vi "serial del.vi"() -> ()   [LabVIEW 2014]
uses:
  <vilib>/Utility/sysdir.llb/System Directory Type.ctl
panel:
  in  "?":bool
  out "?":string
  in  "정규식":string
  in  "정규식 2":string
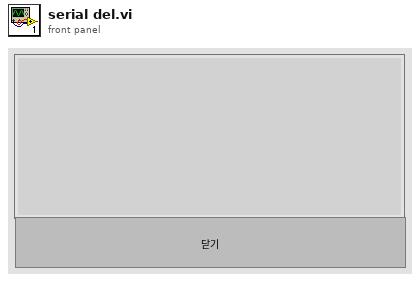
[diagram p1: front panel]
types:
  T1 = enum16{"open", "replace", "create", "open or create", "replace or create", "replace or create with confirmation"}
  T2 = typedef "System Directory Type.ctl" = i32
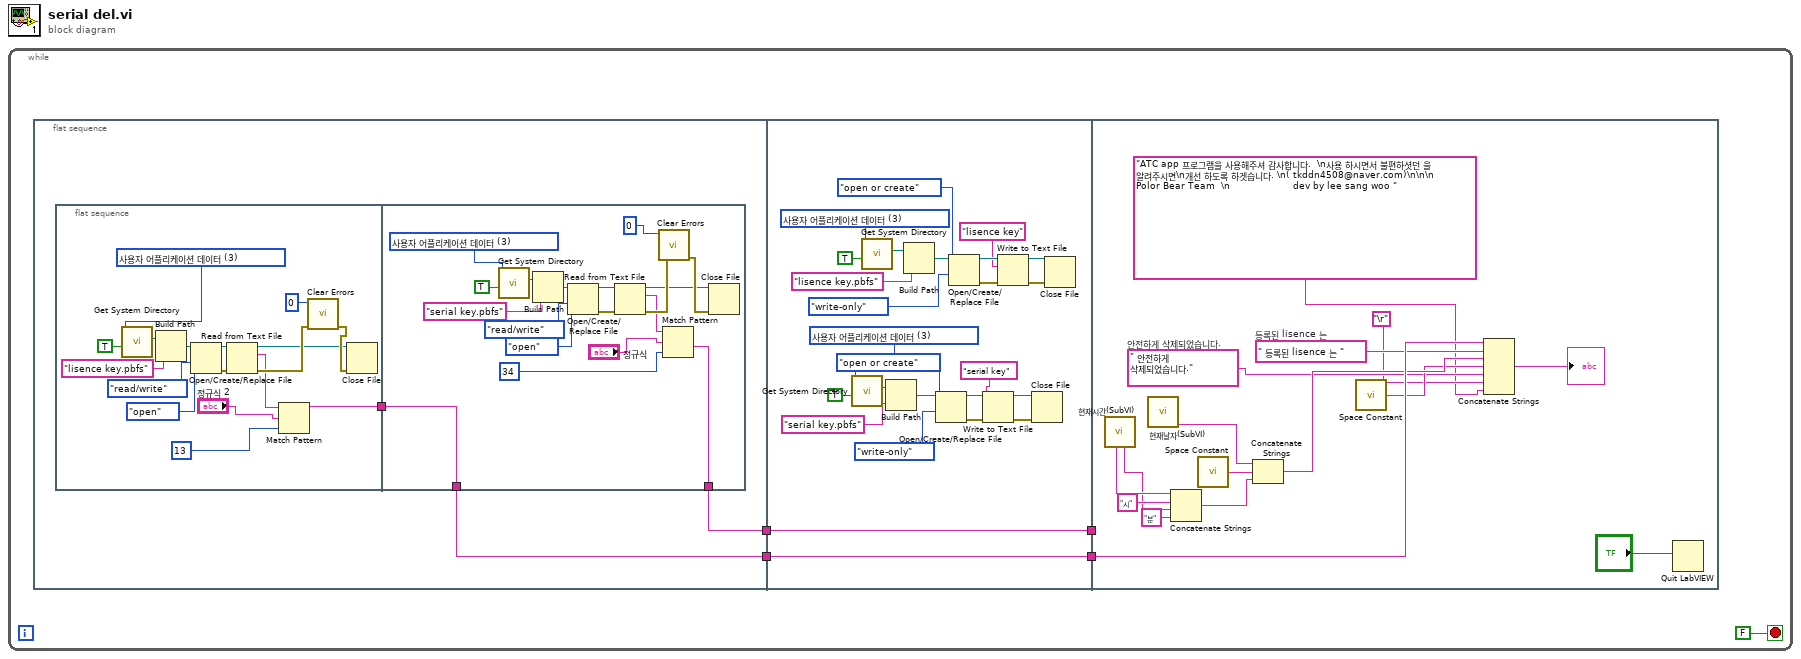
[diagram p0: block diagram]
diagram:
  n1 = while {
    stop <- FALSE stop-if-true
    n2 = flat-sequence {
      tunnel: [w7] -> w5
      tunnel: [w6] -> w4
      tunnel: w5 -> [w44]
      tunnel: [w45] -> w3
      tunnel: w4 -> [w45]
      tunnel: [w44] -> w2
      tunnel: w3 -> [w85]
      tunnel: w2 -> [_]
      frame #0 {
        n3 = flat-sequence {
          tunnel: [w10] -> w8
          tunnel: w8 -> [w27]
          tunnel: [w28] -> w7
          tunnel: [w27] -> w6
          frame #0 {
            w15 = T2 3 items=["사용자 홈"=0, "사용자 데스크탑"=1, "사용자 문서"=2, "사용자 어플리케이션 데이터"=3, "사용자 환경"=4, "사용자 임시"=5, "퍼블릭 문서"=6, "퍼블릭 어플리케이션 데이터"=7, "퍼블릭 환경"=8, "퍼블릭 캐시"=13, "시스템 코어 라이브러리"=9, "시스템 설치된 라이브러리"=10, "어플리케이션 파일"=11, "부팅 볼륨 루트"=12] ("system directory type")
            n4 = call <vilib>:"Get System Directory.vi"("create directory if not found? (F)"=TRUE, "system directory type"=w15) -> ("system directory"=w14:path)  [unwired: 9 in]
            n5 = Build Path(base path=w14, name or relative path="lisence key.pbfs" ("이름 또는 상대 경로")) -> (appended path=w13:path)
            n6 = Open/Create/Replace File(file path (use dialog)=w13, operation (0:open)=T1."open" ("동작(0:open)"), access (0:read/write)=enum16{"read/write", "read-only", "write-only"}."read/write" ("접근(0:읽기/쓰기)")) -> (refnum out=w19:refnum<file>, error out=w18:errorcluster)  [unwired: 3 in, 1 out]
            n7 = Read from Text File(file (use dialog)=w19, error in=w18) -> (refnum out=w20:refnum<file>, text=w21:string, error out=w23:errorcluster)  [unwired: 2 in, 1 out]
            n8 = Match Pattern(string=w21, regular expression="정규식 2", offset (0)=13 ("오프셋(0) 2")) -> (before substring=w10:string)  [unwired: 3 out]
            n9 = call <vilib>:"Clear Errors.vi"("error in (no error)"=w23, "specific error code to clear (0: all)"=0) -> ("error out"=w24:errorcluster)  [unwired: 4 in, 1 out]
            n10 = Close File(refnum=w20, error in=w24) -> ()  [unwired: 2 out]
          }
          frame #1 {
            w36 = T2 3 items=["사용자 홈"=0, "사용자 데스크탑"=1, "사용자 문서"=2, "사용자 어플리케이션 데이터"=3, "사용자 환경"=4, "사용자 임시"=5, "퍼블릭 문서"=6, "퍼블릭 어플리케이션 데이터"=7, "퍼블릭 환경"=8, "퍼블릭 캐시"=13, "시스템 코어 라이브러리"=9, "시스템 설치된 라이브러리"=10, "어플리케이션 파일"=11, "부팅 볼륨 루트"=12] ("system directory type")
            n11 = call <vilib>:"Get System Directory.vi"("create directory if not found? (F)"=TRUE, "system directory type"=w36) -> ("system directory"=w37:path)  [unwired: 9 in]
            n12 = Build Path(base path=w37, name or relative path="serial key.pbfs" ("이름 또는 상대 경로")) -> (appended path=w38:path)
            n13 = Open/Create/Replace File(file path (use dialog)=w38, operation (0:open)=T1."open" ("동작(0:open)"), access (0:read/write)=enum16{"read/write", "read-only", "write-only"}."read/write" ("접근(0:읽기/쓰기)")) -> (refnum out=w32:refnum<file>, error out=w33:errorcluster)  [unwired: 3 in, 1 out]
            n14 = Read from Text File(file (use dialog)=w32, error in=w33) -> (refnum out=w31:refnum<file>, text=w39:string, error out=w41:errorcluster)  [unwired: 2 in, 1 out]
            n15 = call <vilib>:"Clear Errors.vi"("error in (no error)"=w41, "specific error code to clear (0: all)"=0) -> ("error out"=w42:errorcluster)  [unwired: 4 in, 1 out]
            n16 = Match Pattern(string=w39, regular expression="정규식", offset (0)=34 ("오프셋(0)")) -> (after substring=w28:string)  [unwired: 3 out]
            n17 = Close File(refnum=w31, error in=w42) -> ()  [unwired: 2 out]
          }
        }
      }
      frame #1 {
        w53 = T2 3 items=["사용자 홈"=0, "사용자 데스크탑"=1, "사용자 문서"=2, "사용자 어플리케이션 데이터"=3, "사용자 환경"=4, "사용자 임시"=5, "퍼블릭 문서"=6, "퍼블릭 어플리케이션 데이터"=7, "퍼블릭 환경"=8, "퍼블릭 캐시"=13, "시스템 코어 라이브러리"=9, "시스템 설치된 라이브러리"=10, "어플리케이션 파일"=11, "부팅 볼륨 루트"=12] ("system directory type")
        w65 = T2 3 items=["사용자 홈"=0, "사용자 데스크탑"=1, "사용자 문서"=2, "사용자 어플리케이션 데이터"=3, "사용자 환경"=4, "사용자 임시"=5, "퍼블릭 문서"=6, "퍼블릭 어플리케이션 데이터"=7, "퍼블릭 환경"=8, "퍼블릭 캐시"=13, "시스템 코어 라이브러리"=9, "시스템 설치된 라이브러리"=10, "어플리케이션 파일"=11, "부팅 볼륨 루트"=12] ("system directory type")
        n18 = call <vilib>:"Get System Directory.vi"("create directory if not found? (F)"=TRUE, "system directory type"=w65) -> ("system directory"=w66:path)  [unwired: 9 in]
        n19 = call <vilib>:"Get System Directory.vi"("create directory if not found? (F)"=TRUE, "system directory type"=w53) -> ("system directory"=w52:path)  [unwired: 9 in]
        n20 = Build Path(base path=w66, name or relative path="serial key.pbfs" ("이름 또는 상대 경로")) -> (appended path=w67:path)
        n21 = Build Path(base path=w52, name or relative path="lisence key.pbfs" ("이름 또는 상대 경로")) -> (appended path=w51:path)
        n22 = Open/Create/Replace File(file path (use dialog)=w67, operation (0:open)=T1."open or create" ("동작(0:open)"), access (0:read/write)=enum16{"read/write", "read-only", "write-only"}."write-only" ("접근(0:읽기/쓰기)")) -> (refnum out=w60:refnum<file>, error out=w61:errorcluster)  [unwired: 3 in, 1 out]
        n23 = Open/Create/Replace File(file path (use dialog)=w51, operation (0:open)=T1."open or create" ("동작(0:open)"), access (0:read/write)=enum16{"read/write", "read-only", "write-only"}."write-only" ("접근(0:읽기/쓰기)")) -> (refnum out=w55:refnum<file>, error out=w56:errorcluster)  [unwired: 3 in, 1 out]
        n24 = Write to Text File(file (use dialog)=w60, text="serial key" ("이름 또는 상대 경로"), error in=w61) -> (refnum out=w63:refnum<file>, error out=w62:errorcluster)  [unwired: 1 in, 1 out]
        n25 = Write to Text File(file (use dialog)=w55, text="lisence key" ("이름 또는 상대 경로"), error in=w56) -> (refnum out=w54:refnum<file>, error out=w57:errorcluster)  [unwired: 1 in, 1 out]
        n26 = Close File(refnum=w63, error in=w62) -> ()  [unwired: 2 out]
        n27 = Close File(refnum=w54, error in=w57) -> ()  [unwired: 2 out]
      }
      frame #2 {
        w77 = " 등록된 lisence 는 "  # 등록된 lisence 는
        w74 = " 안전하게 삭제되었습니다."  # 안전하게 삭제되었습니다.
        n28 = call "현재시간(SubVI).vi"() -> ("분 문자열"=w82:string, "시 문자열"=w84:string)  [unwired: 3 in, 7 out]
        n29 = call "현재날자(SubVI).vi"() -> ("월,일 을 문자열로"=w78:string)  [unwired: 5 in, 6 out]
        n30 = Concatenate Strings(w84, "시", w82, "분" ("문자열")) -> (w80:string)
        n31 = call <vilib>:"Space Constant.vi"() -> ("String"=w79:string)
        n32 = Concatenate Strings(w78, w79, w80) -> (w76:string)
        n33 = call <vilib>:"Space Constant.vi"() -> ("String"=w75:string)
        n34 = Concatenate Strings(w85, w77, w76, w75, w74, "\r", "ATC app 프로그램을 사용해주셔 감사합니다.  \n사용 하시면서 불편하셧던 을 알려주시면\n개선 하도록 하겟습니다. \n( tkddn4508@naver.com)\n\n\n                           Polor Bear Team  \n                     dev by lee sang woo " ("Message")) -> (→"?":string)
        n35 = Quit LabVIEW(quit? (T)="?") -> ()
      }
    }
  }
